vi "Write fpgaSession.vi"(8 "error in (no error)":errorcluster, 10 "Session Handle":T1, 11 "FPGA Serial Session in":refnum<class "FPGA Serial Session.lvclass">) -> (0 "error out":errorcluster, 3 "FPGA Serial Session out":refnum<class "FPGA Serial Session.lvclass">)   [LabVIEW 2014, in "FPGA Serial Session.lvclass"]
uses:
  FPGA Serial Session.lvclass
  <userlib>/_Session Fwk/Typedefs/Session Handle.ctl
  <userlib>/_Session Fwk/Session - Root.lvclass
  FPGA Serial Session.lvclass/FPGA Serial Session.ctl
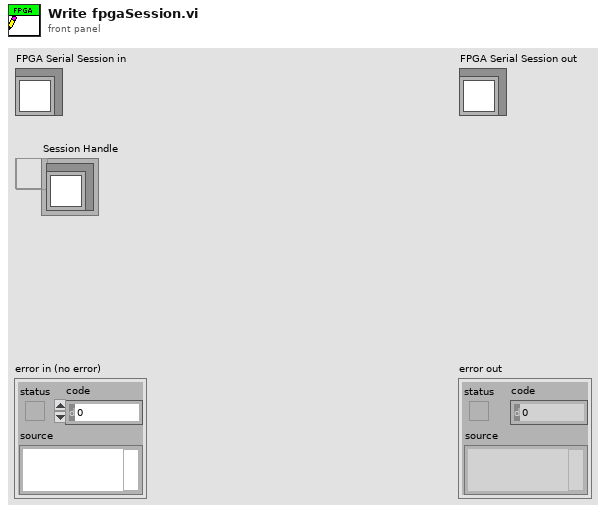
[diagram p1: front panel]
types:
  T1 = typedef "Session - Root.lvclass/Session Handle.ctl" = refnum<data-value>
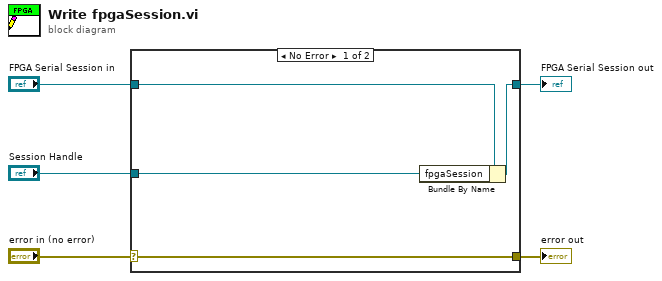
[diagram p0: block diagram]
diagram:
  n1 = case shown="No Error" "error in (no error)" {
    selector: "error in (no error)" -> [w9 w10]
    tunnel: [w9 w10] -> w4
    tunnel: [w7 w11] -> w2
    tunnel: "FPGA Serial Session in" -> [w8 w11]
    tunnel: "Session Handle" -> [w6 _]
    frame No Error {
      n2 = Bundle By Name(cluster=w8, "fpgaSession"=w6) -> (w7:refnum<class "FPGA Serial Session.lvclass">)
    }
    frame Error {
    }
  }
  "error out" <- w4
  "FPGA Serial Session out" <- w2
